vi "AttentuationToTheta.vi"(0 "Attentuation [dB]":i32) -> (1 "abs(theta)":dbl, 2 "sign":i32)   [LabVIEW 2018]
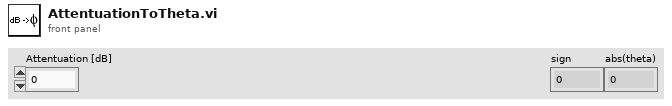
[diagram p1: front panel]
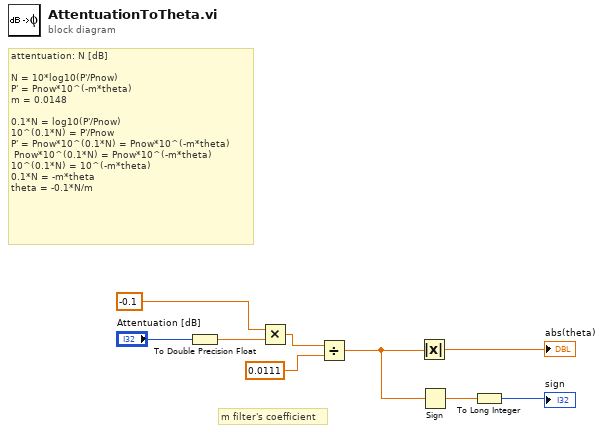
[diagram p0: block diagram]
diagram:
  # "m filter's coefficient"
  # "attentuation: N [dB]\n\nN = 10*log10(P'/Pnow)\nP' = Pnow*10^(-m*theta)\nm = 0.0148\n\n0.1*N = log10(P'/Pnow)\n10^(0.1*N) = P'/Pnow\nP' = Pnow*10^(0.1*N) = Pnow*10^(-m*theta)\n Pnow*10^(0.1*N) = Pnow*10^(-m*theta)\n10^(0.1*N) = 10^(-m*theta)\n0.1*N = -m*theta\ntheta = -0.1*N/m"
  n1 = To Double Precision Float(number="Attentuation [dB]") -> (double precision float=w1:dbl)
  n2 = Multiply(x=-0.1, y=w1) -> (x*y=w9:dbl)
  n3 = Divide(x=w9, y=0.0111) -> (x/y=w6:dbl)
  n4 = Absolute Value(x=w6) -> (abs(x)=→"abs(theta)":dbl)
  n5 = Sign(1:w6) -> (0:w4:dbl)
  n6 = To Long Integer(number=w4) -> (32bit integer=→"sign":i32)
